vi "SciScript_coMD.vi"() -> ()   [LabVIEW 2012]
doc: "SciScan 1.2 160622"
panel:
  out "stripped path":path
  out "error out":errorcluster
  out "Application:Directory Path":path
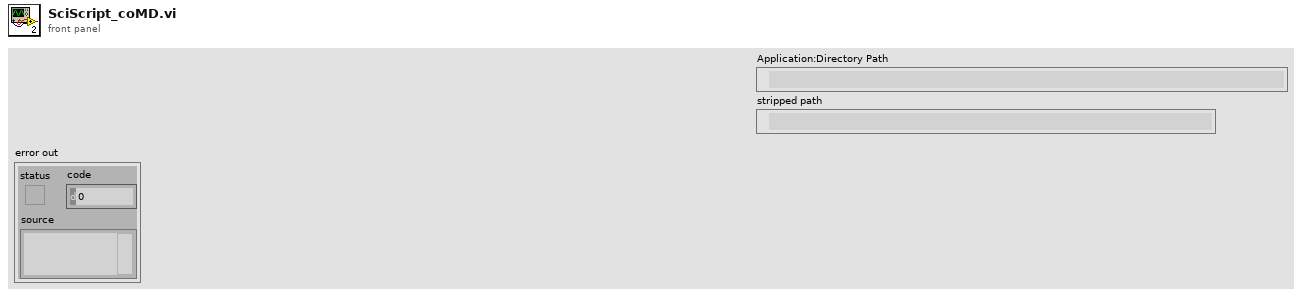
[diagram p1: front panel]
types:
  T1 = enum32{"Invalid", "Standard", "Closed", "Hidden", "Minimized", "Maximized"}
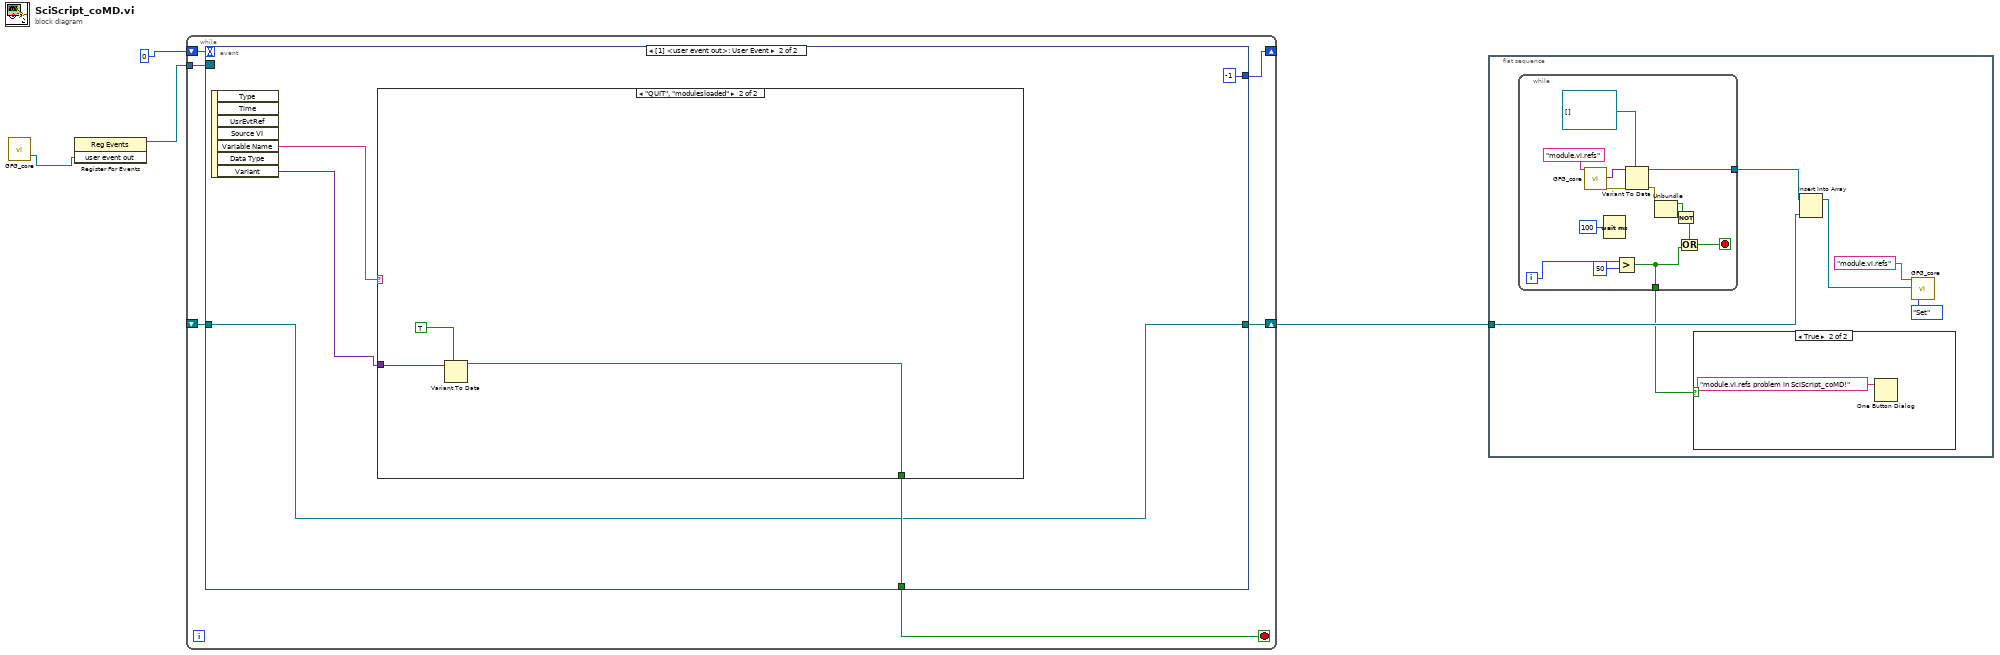
[diagram p0: block diagram]
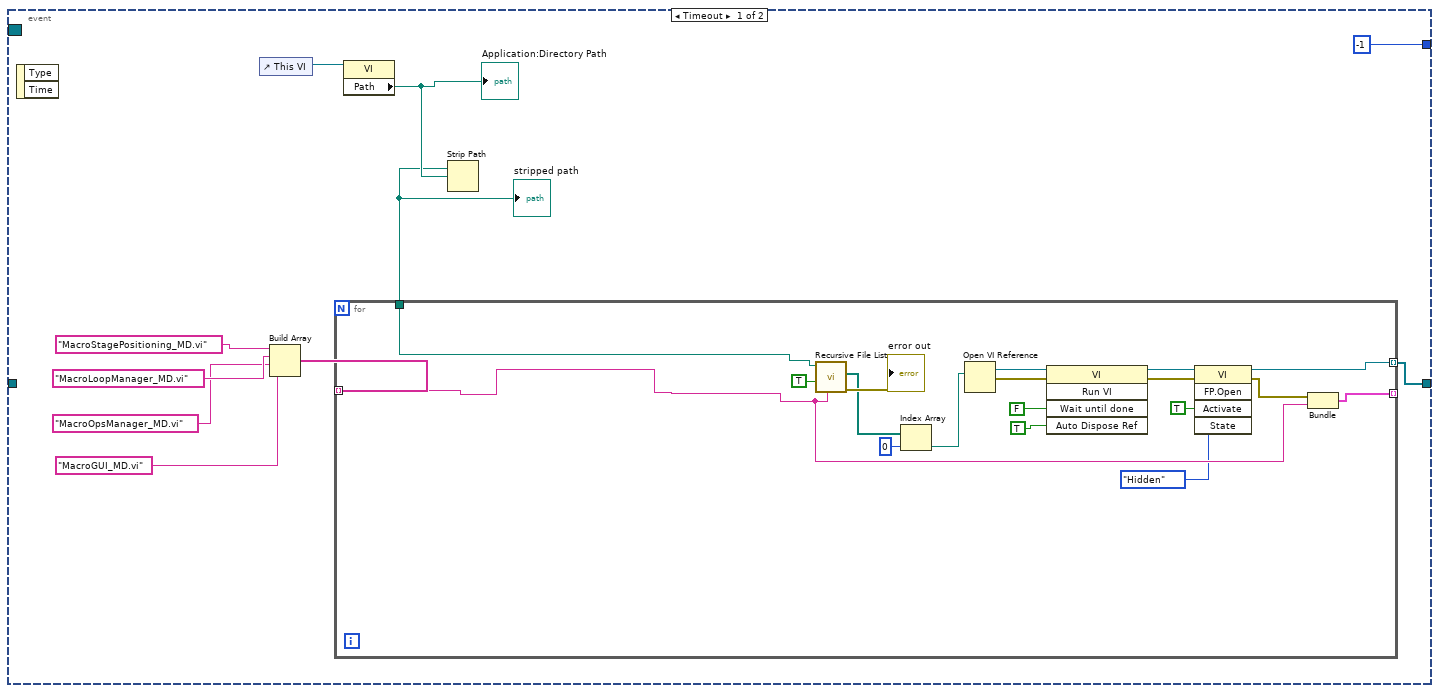
[diagram p3: hidden frame]
diagram:
  n1 = call "GFG_core.vi"() -> ("user event out"=w3:refnum<user-event>)  [unwired: 13 in, 6 out]
  n2 = register-events(w3) -> (reference out=w2:refnum<event-registration>)  [unwired: 2 in, 1 out]
  n3 = while {
    tunnel: w2 -> [w9]
    shift-right: [w10] -> w4
    shift-left: _ -> [w6]
    shift-right: [w5] -> _
    shift-left: 0 -> [w8]
    stop <- w7 stop-if-true
    n4 = event shown="[1] <user event out>: User Event" {
      selector: w9 -> [_ _]
      dyn-events: _ -> [_ _]
      timeout: w8 -> [_ _]
      tunnel: [w12 w41] -> w10
      tunnel: [_ w42] -> w7
      tunnel: w6 -> [_ w41]
      tunnel: [-1 -1] -> w5
      event Timeout {
        n5 = event-data() -> ()  [unwired: 1 in, 2 out]
        n6 = control-ref of="This VI"() -> (w20:refnum<vi>)
        n7 = Build Array("MacroStagePositioning_MD.vi", "MacroLoopManager_MD.vi", "MacroOpsManager_MD.vi", "MacroGUI_MD.vi") -> (w15:string[])
        n8 = property class="VI"(reference=w20) -> ("Path"=w14:path)  [unwired: 1 in, 2 out]
        "Application:Directory Path" <- w14
        n9 = Strip Path(path=w14) -> (stripped path=w13:path)  [unwired: 1 out]
        "stripped path" <- w13
        n10 = for {
          tunnel: w15 -> [w36] mode=indexing
          tunnel: [w38] -> w12 mode=indexing
          tunnel: w13 -> [w35]
          tunnel: [w37] -> _ mode=indexing
          n11 = call <vilib>:"Recursive File List.vi"("pattern"=w36, "Continue Recursing on Error? (F)"=TRUE, "Folder Path"=w35) -> ("error out"=→"error out":errorcluster, "All Files in Dir"=w32:path[])  [unwired: 4 in, 3 out]
          n12 = Index Array(array=w32, index=0) -> (element=w21:path)
          n13 = Open VI Reference(vi path=w21) -> (vi reference=w25:refnum<vi>, error out=w30:errorcluster)  [unwired: 5 in]
          n14 = invoke class="VI" method="Run VI"(reference=w25, error in=w30, "Wait until done"=FALSE, "Auto Dispose Ref"=TRUE ("Auto Dispose Reference")) -> (reference out=w23:refnum<vi>, error out=w28:errorcluster)  [unwired: 1 in, 3 out]
          n15 = invoke class="VI" method="FP.Open"(reference=w23, error in=w28, "Activate"=TRUE ("Activate?"), "State"=T1."Hidden") -> (reference out=w38:refnum<vi>, error out=w29:errorcluster)  [unwired: 1 in, 3 out]
          n16 = Bundle("error out"=w29, w36) -> (w37:cluster{"error out":errorcluster, string})  [unwired: 1 in]
        }
      }
      event User Event {
        n17 = event-data() -> ("Variable Name"=w43:string, "Variant"=w39:variant)  [unwired: 1 in, 5 out]
        n18 = case shown="\"QUIT\", \"modulesloaded\"" w43 {
          tunnel: [_ w44] -> w42
          tunnel: w39 -> [_ w46]
          frame "False", Default {
          }
          frame "QUIT", "modulesloaded" {
            n19 = Variant To Data(type=TRUE, Variant=w46) -> (data=w44:bool)  [unwired: 1 in, 1 out]
          }
        }
      }
    }
  }
  n20 = flat-sequence {
    tunnel: w4 -> [w48]
    frame #0 {
      n21 = while {
        tunnel: [w66] -> w50
        tunnel: [w54] -> w47
        i -> [w60]
        stop <- w55 stop-if-true
        n22 = call "GFG_core.vi"("Variable Name in"="module.vi.refs") -> ("Variant Out"=w64:variant, "error out"=w63:errorcluster)  [unwired: 12 in, 5 out]
        n23 = Wait (ms)(milliseconds to wait=u32 100) -> ()  [unwired: 1 out]
        n24 = Greater?(x=w60, y=50) -> (0:w54:bool)
        n25 = Variant To Data(error in=w63, type=refnum<vi>[] [], Variant=w64) -> (data=w66:refnum<vi>[], error out=w58:errorcluster)
        n26 = Unbundle(w58) -> ("status"=w57:bool)  [unwired: 2 out]
        n27 = Not(x=w57) -> (.not. x?=w56:bool)
        n28 = Or(x=w56, y=w54) -> (x .or. y?=w55:bool)
      }
      n29 = case shown="True" w47 {
        frame False {
        }
        frame True {
          n30 = One Button Dialog(message="module.vi.refs problem in SciScript_coMD!") -> ()  [unwired: 1 in, 1 out]
        }
      }
      n31 = Insert Into Array(array=w50, new element=w48) -> (w52:refnum<vi>[])  [unwired: 1 in]
      n32 = call "GFG_core.vi"("Variable Name in"="module.vi.refs", "Variant in"=w52, "Action"=enum16{"Init", "Set", "Get"}."Set") -> ()  [unwired: 10 in, 7 out]
    }
  }
